vi "Get Devices.vi"(8 "error in (no error)":errorcluster, 11 "Agilis in":T1) -> (0 "error out":errorcluster, 2 "Devices":string[](array[string]), 3 "Agilis out":T1)   [LabVIEW 2016, in "Drivers.lvlib" / "Agilis.lvlib"]
uses:
  Agilis.lvlib
  AgilisCmdLib Refnum.ctl
  Z:/TraceGrabber/Drivers/Agilis/AgilisCmdLib.dll
  AgilisCmdLib.dll
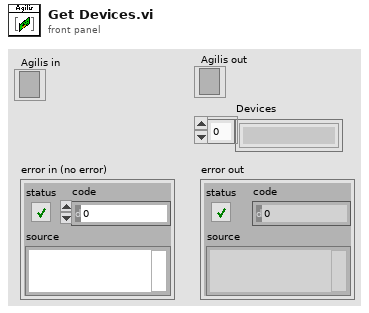
[diagram p1: front panel]
types:
  T1 = typedef "Drivers.lvlib/Agilis.lvlib/AgilisCmdLib Refnum.ctl" = refnum<k24>
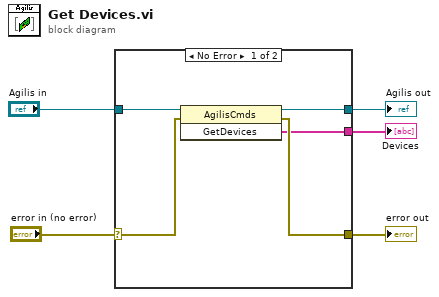
[diagram p0: block diagram]
diagram:
  n1 = case shown="No Error" "error in (no error)" {
    selector: "error in (no error)" -> [w9 w12]
    tunnel: "Agilis in" -> [w10 w11]
    tunnel: [w8 w11] -> w3
    tunnel: [w7 w12] -> w2
    tunnel: [w6 _] -> w1
    frame No Error {
      n2 = invoke class="AgilisCmds" method="GetDevices"(reference=w10, error in=w9) -> (reference out=w8:T1, error out=w7:errorcluster, "GetDevices"=w6:string[])  [unwired: 1 in]
    }
    frame Error {
    }
  }
  "Agilis out" <- w3
  "error out" <- w2
  "Devices" <- w1
